vi "CenterFinderUsing2Points.vi"(0 "Operation":enum16{"Manual", "DrawCircle", "Automatic"}(ring)=enum."DrawCircle", 1 "Zone":enum16{"ZoneA", "ZoneB", "ZoneC", "ZoneD"}(ring), 2 "Autofocus":T3={"Enable"=TRUE, "InitialStepSize"=0.05, "Tolerance"=0.02, "Abort"=FALSE} {"Tolerance" format="%#_13g"}, 5 "Component":enum16{"BP", "Si", "HB", "HBonBP", "Other"}(ring), 7 "StopJoyStick":bool, 9 "VisibilityInCamera":enum16{"JoyStick", "AllVisible"}(ring)=enum."AllVisible", 11 "error in (no error)":errorcluster, 12 "Position":enum16{"1", "2"}(ring), 13 "SaveImagesLog":bool=TRUE) -> (4 "Output XYZU":string, 6 "Image":T4(plugin-control), 8 "Image 2":T4[](array[plugin-control]) caption="AllImages", 15 "error out":errorcluster)   [LabVIEW 2021]
uses:
  <vilib>/userDefined/High Color/IMAQdx.ctl
  <vilib>/Analysis/coordinate.llb/2D Cartesian Coordinate Rotation (Scalar).vi
  <vilib>/Analysis/baseanly.llb/Mean (DBL).vi
  include/GlobalVariables.vi
  Other Models/2010/Motion/AbortSingle.vi
  <vilib>/Analysis/NI_AALPro.lvlib
  <vilib>/Analysis/NI_AALBase.lvlib
  <vilib>/vision/driver/NI_Vision_Acquisition_Software.lvlib
panel:
  in  "YoffsetMidFid":dbl=3.5005
  in  "XoffsetMidFid":dbl
  out "DistFids":dbl=50.0
  out "AllMatches":T1(array[cluster]) {"Bounding Box"."y" format="%.2f"; "Bounding Box"."x" format="%.2f"; "Score" format="%.2f"; "Scale" format="%.2f"; "Angle" format="%.2f"; "Position"."y" format="%.2f"; "Position"."x" format="%.2f"}
  in  "Camera":T2="cam1"
  out "OutputFile":string
  out "spreadsheet string 2":string
  out "spreadsheet string":string
  in  "ModuleName":string="T1"
  out "SyringeY":dbl format="%#_7g"
  out "SyringeX":dbl format="%#_7g"
  in  "CamToSyringeYoffset":dbl=126.651
  in  "CamToSyringeXoffset":dbl=167.702
  out "FileUsedForFiducials":string
  out "UsedCoordinates":string
  out "CameraGcode":string
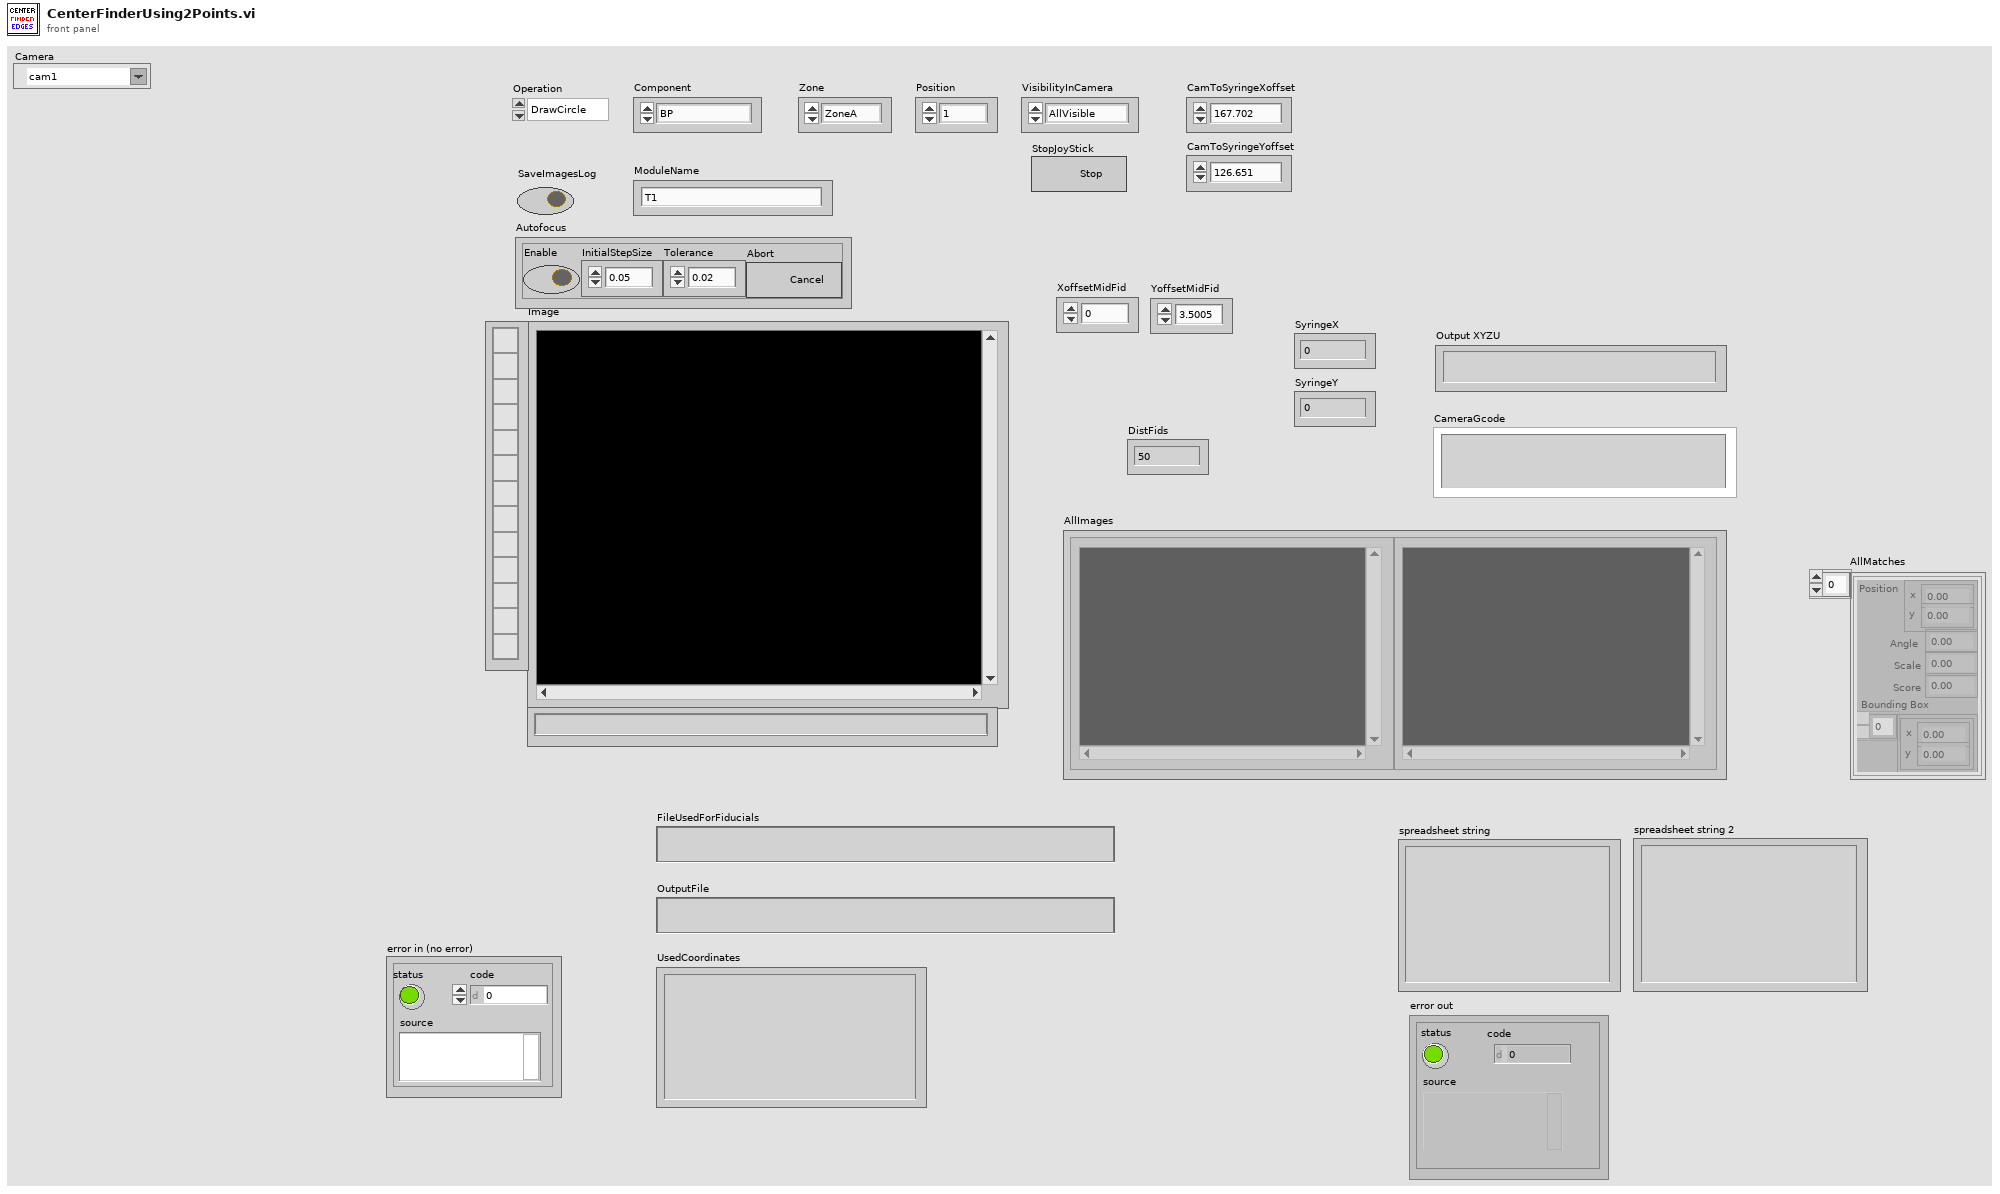
[diagram p1: front panel]
types:
  T1 = cluster{"Position":cluster{"x":sgl, "y":sgl}, "Angle":sgl, "Scale":sgl, "Score":sgl, "Bounding Box":cluster{"x":sgl, "y":sgl}[]}[]
  T2 = typedef "IMAQdx.ctl" = refnum<k21>
  T3 = cluster{"Enable":bool, "InitialStepSize":dbl, "Tolerance":dbl, "Abort":bool}
  T4 = typedef "IMAQ Image.ctl" = refnum<image>
  T5 = cluster{"Number of Matches Requested":i32, "Minimum Match Score":sgl, "Angle Ranges":cluster{"Start Angle":sgl, "End Angle":sgl}[]}
  T6 = typedef "Image Type" = u32
  T7 = typedef "IMAQ Point" = cluster{"X":sgl, "Y":sgl}
  T8 = typedef "IMAQ Circle" = cluster{"Center X":i32, "Center Y":i32, "Inner Radius":i32, "Outer Radius":i32, "Start Angle":dbl, "End Angle":dbl}
  T9 = enum16{"Left Button", "Center Button", "Right Button", "Window Close"}
  T10 = enum16{"open", "replace", "create", "open or create", "replace or create", "replace or create with confirmation"}
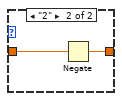
[diagram p2: hidden frame]
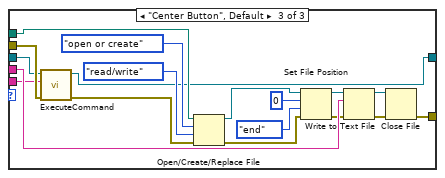
[diagram p5: hidden frame]
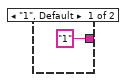
[diagram p6: hidden frame]
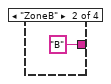
[diagram p7: hidden frame]
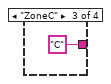
[diagram p8: hidden frame]
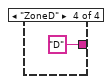
[diagram p9: hidden frame]
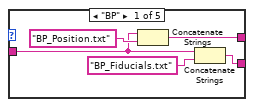
[diagram p10: hidden frame]
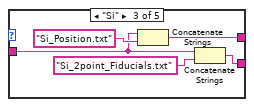
[diagram p11: hidden frame]
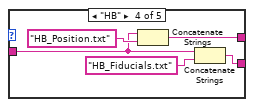
[diagram p12: hidden frame]
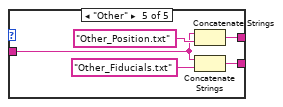
[diagram p13: hidden frame]
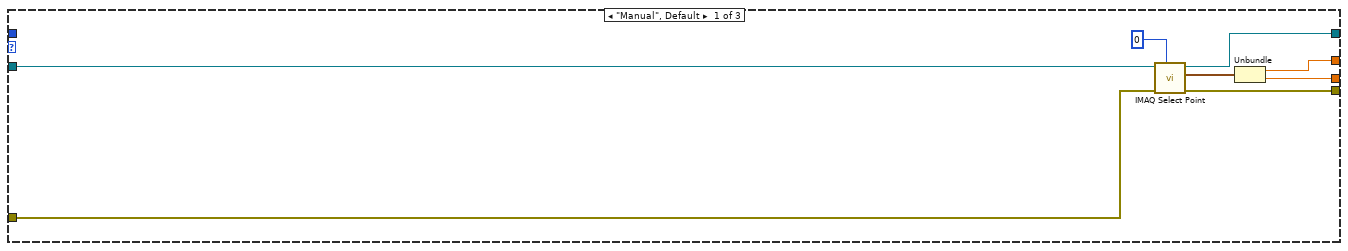
[diagram p14: hidden frame]
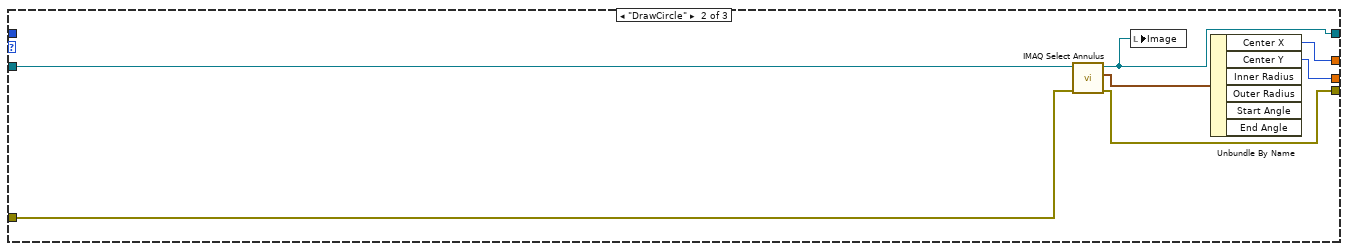
[diagram p15: hidden frame]
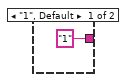
[diagram p17: hidden frame]
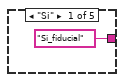
[diagram p18: hidden frame]
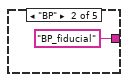
[diagram p19: hidden frame]
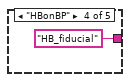
[diagram p20: hidden frame]
diagram:
  w49 = "%f" ("format string")
  w87 = "\t"
  w84 = i16 6 ("width (-)")
  # "Write the XYZU of the baseplate to a text file & move the gantry?"
  # "Prepare to move the gantry to see the center of baseplate in camera."
  # "AllVisble: Assumes that you know the coordinates of all corners (fiducials) well. No need for any adjustments.\nJoyStick: Use joystick at each point to make good image.\nClickMove: Use \"AdjustCamera\" panel and move the gantry stepwise. Click \"Done\" when you're satisfied with the picture."
  n1 = flat-sequence {
    tunnel: [w96] -> w45
    tunnel: w45 -> [w112]
    tunnel: [w111] -> w44
    tunnel: [w110] -> w42
    tunnel: [w109] -> w39
    tunnel: w44 -> [w164]
    tunnel: [w164] -> w43
    tunnel: w42 -> [w157]
    tunnel: [w152] -> w41
    tunnel: [w163] -> w40
    tunnel: w39 -> [w162]
    tunnel: [w162] -> w38
    tunnel: [w156] -> w30
    tunnel: [w155] -> w29
    tunnel: 2 -> [w191]
    tunnel: "VisibilityInCamera" -> [w184]
    tunnel: w43 -> [w182]
    tunnel: w41 -> [w174]
    tunnel: w40 -> [w181]
    tunnel: w38 -> [w180]
    tunnel: w30 -> [w172]
    tunnel: w29 -> [w173]
    tunnel: [w190] -> w28
    tunnel: [w189] -> w27
    tunnel: [w188] -> w26
    tunnel: [w187] -> w25
    tunnel: [w186] -> w24
    tunnel: [w185] -> w23
    tunnel: [w183] -> w22
    tunnel: [w180] -> w21
    tunnel: [w179] -> w20
    tunnel: [w171] -> w19
    tunnel: [w468] -> w36
    tunnel: [w469] -> w37
    tunnel: [w470] -> w54
    tunnel: [w471] -> w15
    tunnel: [w465] -> w16
    tunnel: [w472] -> _
    tunnel: [w473] -> w91
    tunnel: [w474] -> w50
    tunnel: [w475] -> w51
    tunnel: w28 -> [w475]
    tunnel: w27 -> [w474]
    tunnel: w26 -> [w473]
    tunnel: w25 -> [w472]
    tunnel: w24 -> [w466]
    tunnel: w23 -> [w471]
    tunnel: w22 -> [w470]
    tunnel: w21 -> [w469]
    tunnel: w20 -> [w468]
    tunnel: w19 -> [w467]
    frame #0 {
      n2 = case shown="\"ZoneA\", Default" "Zone" {
        tunnel: ["A" "B" "C" "D"] -> w100
        frame "ZoneA", Default {
        }
        frame "ZoneB" {
        }
        frame "ZoneC" {
        }
        frame "ZoneD" {
        }
      }
      n3 = case shown="\"2\"" "Position" {
        tunnel: ["1" "2"] -> w101
        frame "1", Default {
        }
        frame "2" {
        }
      }
      n4 = Concatenate Strings(w100, w101, "_" ("string")) -> (w96:string)
      "UsedCoordinates" <- ""
    }
    frame #1 {
      n5 = Concatenate Strings("C:\\Users\\TTUHEP\\Documents\\LabVIEW\\GantryPrograms\\", "Configs\\" ("string"), w112) -> (w119:string)
      n6 = case shown="\"HBonBP\"" "Component" {
        tunnel: w119 -> [w127 w132 w138 w143 w148]
        tunnel: [w128 w133 w140 w145 w150] -> w122
        tunnel: [w129 w134 w137 w142 w147] -> w109
        frame "BP" {
          n7 = Concatenate Strings(w127, "BP_Position.txt") -> (w129:string)
          n8 = Concatenate Strings(w127, "BP_Fiducials.txt") -> (w128:string)
        }
        frame "HBonBP" {
          n9 = Concatenate Strings(w132, "BP_Position.txt") -> (w134:string)
          n10 = Concatenate Strings(w132, "HBonBP_Fiducials.txt") -> (w133:string)
        }
        frame "Si" {
          n11 = Concatenate Strings(w138, "Si_Position.txt") -> (w137:string)
          n12 = Concatenate Strings(w138, "Si_2point_Fiducials.txt") -> (w140:string)
        }
        frame "HB" {
          n13 = Concatenate Strings(w143, "HB_Position.txt") -> (w142:string)
          n14 = Concatenate Strings(w143, "HB_Fiducials.txt") -> (w145:string)
        }
        frame "Other" {
          n15 = Concatenate Strings(w148, "Other_Position.txt") -> (w147:string)
          n16 = Concatenate Strings(w148, "Other_Fiducials.txt") -> (w150:string)
        }
      }
      "FileUsedForFiducials" <- w122
      "OutputFile" <- w109
      n17 = String To Path(string=w122) -> (path=w120:path)
      n18 = Concatenate Strings("This file does not exist:" ("ErrorMessage"), w122) -> (w123:string)
      n19 = call <vilib>:"Check if File or Folder Exists.vi"("error in (no error)"="error in (no error)", "path"=w120) -> ("error out"=w121:errorcluster, "file or folder exists?"=w124:bool, "dup path"=w111:path)  [unwired: 7 in]
      n20 = Not(x=w124) -> (.not. x?=w125:bool)
      n21 = call "AddError.vi"("NoErrorMessage"="InFile OK", "ErrorMessage"=w123, "error in"=w121, "code"=-995, "Error?"=w125) -> ("Error out"=w110:errorcluster)  [unwired: 6 in]
    }
    frame #2 {
      w158 = T6 0 items=["Grayscale (U8)", "Grayscale (I16)", "Grayscale (SGL)", "Complex (CSG)", "RGB (U32)", "HSL (U32)", "RGB (U64)", "Grayscale (U16)"] ("Image Type")
      # "Set the size of the window while selecting the point."
      n22 = call "IMAQ WindSize"("Scrollbars? (N)"=TRUE, "Width & Height"=cluster{"Width":i32, "Height":i32} {"Width"=1333, "Height"=1000}, "Window Number"=0) -> ()  [unwired: 3 in, 3 out]
      n23 = call "IMAQ Create"("Image Name"="name1" ("ImageName"), "Image Type"=w158, "error in (no error)"=w157) -> ("New Image"=w155:T4, "error out"=w160:errorcluster)  [unwired: 2 in]
      n24 = call "Connect.vi"("error in (no error)"=w157) -> ("error out"=w166:errorcluster, "controller"=w167:refnum<k24>)  [unwired: 9 in]
      n25 = call "ExecuteCommand.vi"("error in (no error)"=w166, "Command Code"="G90\nG1 Z0 F100", "controller in"=w167) -> ("error out"=w154:errorcluster, "controller out"=w163:refnum<k24>)  [unwired: 6 in, 1 out]
      n26 = call <vilib>:"IMAQdx Open Camera.vi"("error in"=w160, "Session In"="Camera") -> ("error out"=w153:errorcluster, "Session Out"=w156:T2)  [unwired: 8 in]
      n27 = Merge Errors(w154, w153) -> (w152:errorcluster)
    }
    frame #3 {
      n28 = local read "Autofocus"() -> (w178:T3)
      n29 = local read "Autofocus"() -> (w176:T3)
      n30 = Unbundle By Name(w178) -> ("Enable"=w177:bool)
      n31 = Unbundle By Name(w176) -> ("Abort"=w175:bool)
      n32 = for {
        N: w191 -> [_]
        tunnel: w181 -> [w251]
        tunnel: w182 -> [w234]
        tunnel: [w232] -> w190 mode=indexing
        tunnel: [w231] -> w189 mode=indexing
        tunnel: [w230] -> w188 mode=indexing
        tunnel: [w226] -> w187 mode=indexing
        tunnel: [w225] -> w185
        tunnel: w184 -> [w224]
        tunnel: w175 -> [w223]
        tunnel: w177 -> [w222]
        tunnel: [w218] -> w183
        tunnel: [w213] -> w179 mode=indexing
        shift-right: [w216] -> w186
        shift-left: w174 -> [w200]
        tunnel: w173 -> [w199]
        shift-right: [w193] -> w171
        shift-left: w172 -> [w192]
        i -> [w211]
        w202 = T6 6 items=["Grayscale (U8)", "Grayscale (I16)", "Grayscale (SGL)", "Complex (CSG)", "RGB (U32)", "HSL (U32)", "RGB (U64)", "Grayscale (U16)"] ("Image Type")
        # "Array of XY cluser"
        # "Z array"
        # "Y array"
        # "X array"
        # "Read text file line by line. Each line contains X,Y,Z coordinates for the gantry."
        n33 = call "GetArrayFmTxtFile.vi"("error in"=w200, "LineNo."=w211, "TextFile"=w234) -> ("error out"=w233:errorcluster, "Array"=w258:dbl[])
        n34 = Index Array(array=w258, index=0) -> (element=w253:dbl)
        n35 = Index Array(array=w258, index=1) -> (element=w252:dbl)
        n36 = Index Array(array=w258, index=2) -> (element=w254:dbl)
        n37 = call "Move.vi"("X"=w253, "Absolute"=TRUE, "Y"=w252, "Z"=w254, "SpeedXY (mm/s)"=100.0, "SpeedZ (mm/s)"=100.0, "Move Z first"=FALSE) -> ("Position Gcode"=w250:string)  [unwired: 8 in]
        n38 = call "ExecuteCommand.vi"("error in (no error)"=w233, "Command Code"=w250, "controller in"=w251) -> ("error out"=w198:errorcluster, "controller out"=w249:refnum<k24>)  [unwired: 6 in, 1 out]
        n39 = call <vilib>:"IMAQdx Snap2.vi"("error in"=w198, "Image In"=w199, "Session In"=w192) -> ("error out"=w197:errorcluster, "Image Out"=w195:T4, "Session Out"=w196:T2)  [unwired: 6 in]
        n40 = local write "Image"(w195) -> ()
        n41 = case shown="\"JoyStick\", Default" w224 {
          tunnel: w196 -> [w372 w434]
          tunnel: w249 -> [w390 w446]
          tunnel: w197 -> [w388 w447]
          tunnel: [w368 w435] -> w220
          tunnel: [w377 w441] -> w238
          tunnel: [w378 w439] -> w194
          tunnel: w223 -> [w381 w444]
          tunnel: w222 -> [w375 w445]
          tunnel: "name1" ("ImageName") -> [w374 w433]
          tunnel: w195 -> [w371 w432]
          tunnel: [w367 w431] -> w193
          frame "JoyStick", Default {
            # "Use joystick to go to a position where camera sees good image."
            n42 = while {
              tunnel: [w418] -> w369
              tunnel: w390 -> [w424]
              tunnel: [w423] -> w386
              tunnel: [w422] -> w387
              tunnel: w388 -> [w417]
              tunnel: w372 -> [w415]
              tunnel: w371 -> [w414]
              tunnel: [w413] -> w370
              stop <- w419 stop-if-true
              n43 = call <vilib>:"IMAQdx Snap2.vi"("error in"=w417, "Image In"=w414, "Session In"=w415) -> ("error out"=w416:errorcluster, "Image Out"=w418:T4, "Session Out"=w413:T2)  [unwired: 6 in]
              n44 = local write "Image"(w418) -> ()
              n45 = global read "GlobalVariables.vi" "StopJoyStick"() -> (w420:bool)
              n46 = Or(x="StopJoyStick", y=w420) -> (x .or. y?=w419:bool)
              n47 = case shown="False" w419 {
                tunnel: w424 -> [w426 w430]
                tunnel: w416 -> [w425 w429]
                tunnel: [w425 w428] -> w423
                tunnel: [w426 w427] -> w422
                frame False {
                }
                frame True {
                  n48 = call-poly "Abort.vi"("error in (no error)"=w429, "controller in"=w430) -> ("error out"=w428:errorcluster, "controller out"=w427:refnum<k24>)  [unwired: 8 in]
                }
              }
            }
            n49 = global write "GlobalVariables.vi" "StopJoyStick"(FALSE ("StopJoyStick")) -> ()
            n50 = call "ExecuteCommand.vi"("error in (no error)"=w388, "Command Code"="JOYSTICK 2D RESET\nJOYSTICK 2D AXISGROUP 1 Y X\nJOYSTICK 2D AXISGROUP 2 Y Z\nJOYSTICK 2D ON", "controller in"=w390) -> ("error out"=w389:errorcluster)  [unwired: 6 in, 2 out]
            n51 = call <vilib>:"Clear Errors.vi"("error in (no error)"=w389) -> ()  [unwired: 5 in, 2 out]
            n52 = call "GetGantryPosition.vi"("error in (no error)"=w386, "Controller In"=w387) -> ("error out"=w382:errorcluster, "controller out"=w380:refnum<k24>, "Position_XYZ"=w376:string)  [unwired: 3 in, 4 out]
            n53 = case shown="False" w375 {
              tunnel: w382 -> [w396 w412]
              tunnel: w381 -> [_ w405]
              tunnel: w380 -> [w394 w406]
              tunnel: [w395 w410] -> w379
              tunnel: [w396 w409] -> w378
              tunnel: [w394 w408] -> w377
              tunnel: w376 -> [w395 _]
              tunnel: w374 -> [_ _]
              tunnel: w370 -> [w392 w400]
              tunnel: w369 -> [w393 w399]
              tunnel: [w393 w398] -> w368
              tunnel: [w392 w397] -> w367
              frame False {
              }
              frame True {
                n54 = local read "Autofocus"() -> (w403:T3)
                n55 = Unbundle By Name(w403) -> ("InitialStepSize"=w401:dbl, "Tolerance"=w402:dbl)
                n56 = call "Autofocus.vi"("controller in"=w406, "AbortAutoFocus"=w405, "ImageIn"=w399, "SafeMaxZ"=80.0, "InitialStepSize"=w401, "Tolerance"=w402, "error in (no error)"=w412, "SessionIn"=w400) -> ("controller out"=w411:refnum<k24>, "Image"=w398:T4, "Session Out"=w397:T2, "error out"=w407:errorcluster)  [unwired: 2 in, 2 out]
                n57 = local write "Image"(w398) -> ()
                n58 = call "GetGantryPosition.vi"("error in (no error)"=w407, "Controller In"=w411) -> ("error out"=w409:errorcluster, "controller out"=w408:refnum<k24>, "Position_XYZ"=w410:string)  [unwired: 3 in, 4 out]
              }
            }
            n59 = local read "UsedCoordinates"() -> (w384:string)
            n60 = Concatenate Strings(w384, "\r", w379) -> (w385:string)
            n61 = local write "UsedCoordinates"(w385) -> ()
          }
          frame "AllVisible" {
            # "No need to move gantry to take a good pic."
            n62 = case shown="False" w445 {
              tunnel: w444 -> [_ w459]
              tunnel: [w451 w462] -> w440
              tunnel: [w450 w464] -> w442
              tunnel: w447 -> [w451 w463]
              tunnel: w446 -> [w450 w461]
              tunnel: [w449 w458] -> w435
              tunnel: w434 -> [w448 w454]
              tunnel: w433 -> [_ _]
              tunnel: w432 -> [w449 w453]
              tunnel: [w448 w452] -> w431
              frame False {
              }
              frame True {
                n63 = local read "Autofocus"() -> (w457:T3)
                n64 = Unbundle By Name(w457) -> ("InitialStepSize"=w456:dbl, "Tolerance"=w455:dbl)
                n65 = call "Autofocus.vi"("controller in"=w461, "AbortAutoFocus"=w459, "ImageIn"=w453, "SafeMaxZ"=80.0, "InitialStepSize"=w456, "Tolerance"=w455, "error in (no error)"=w463, "SessionIn"=w454) -> ("controller out"=w464:refnum<k24>, "Image"=w458:T4, "Session Out"=w452:T2, "error out"=w462:errorcluster)  [unwired: 2 in, 2 out]
                n66 = local write "Image"(w458) -> ()
              }
            }
            n67 = local read "UsedCoordinates"() -> (w437:string)
            n68 = call "GetGantryPosition.vi"("error in (no error)"=w440, "Controller In"=w442) -> ("error out"=w439:errorcluster, "controller out"=w441:refnum<k24>, "Position_XYZ"=w438:string)  [unwired: 3 in, 4 out]
            n69 = Concatenate Strings(w437, "\r", w438) -> (w436:string)
            n70 = local write "UsedCoordinates"(w436) -> ()
          }
        }
        n71 = case shown="\"Automatic\"" "Operation" {
          tunnel: [w267 w274 w285] -> w246
          tunnel: [w266 w273 w284] -> w245
          tunnel: [w265 w275 w293] -> w244
          tunnel: w194 -> [w264 w270 w309]
          tunnel: w220 -> [w263 w272 w314]
          tunnel: w211 -> [_ _ _]
          tunnel: [w262 w271 w291] -> w212
          frame "Manual", Default {
            n72 = call "IMAQ Select Point"("Window Number (0...15)"=0, "error in (no error)"=w264, "Image In"=w263) -> ("error out"=w265:errorcluster, "Point"=w268:T7, "Image Out (duplicate)"=w262:T4)  [unwired: 5 in, 1 out]
            n73 = Unbundle(w268) -> ("X"=w267:sgl, "Y"=w266:sgl)
          }
          frame "DrawCircle" {
            n74 = call "IMAQ Select Annulus"("error in (no error)"=w270, "Image In"=w272) -> ("error out"=w275:errorcluster, "Annulus"=w276:T8, "Image Out (duplicate)"=w271:T4)  [unwired: 6 in, 1 out]
            n75 = local write "Image"(w271) -> ()
            n76 = Unbundle By Name(w276) -> ("Center X"=w274:i32, "Center Y"=w273:i32)  [unwired: 4 out]
          }
          frame "Automatic" {
            w289 = sgl 50.0 ("y")
            w307 = ""
            n77 = local read "Position"() -> (w296:enum16{"1", "2"})
            n78 = case shown="\"2\"" w296 {
              tunnel: ["1" "2"] -> w295
              frame "1", Default {
              }
              frame "2" {
              }
            }
            n79 = local read "Component"() -> (w311:enum16{"BP", "Si", "HB", "HBonBP", "Other"})
            n80 = case shown="\"HB\"" w311 {
              tunnel: ["Si_fiducial" "BP_fiducial" "HB_fiducial" "HB_fiducial" "Other_fiducial"] -> w310
              tunnel: w295 -> [_ _ _ _ _]
              frame "Si" {
              }
              frame "BP" {
              }
              frame "HB" {
              }
              frame "HBonBP" {
              }
              frame "Other" {
              }
            }
            n81 = Concatenate Strings("Could not parse/find this template file for pattern recognition:" ("ErrorMessage"), w310) -> (w302:string)
            n82 = call "JSONfileReader.vi"("error in"=w309, "Variant"=w307, "ItemName"=w310, "FileIn"=path "C:/Users/TTUHEP/Documents/LabVIEW/GantryPrograms/Configs/PatternRecognTemplateMaps.json" ("PatterRecognTemplateMap")) -> ("error out"=w299:errorcluster, "Data"=w308:variant, "Found"=w305:bool)
            n83 = Not(x=w305) -> (.not. x?=w304:bool)
            n84 = Variant To Data(error in=w299, type=w307, Variant=w308) -> (data=w306:string, error out=w298:errorcluster)
            n85 = call "AddError.vi"("NoErrorMessage"="Template file name found from json.", "ErrorMessage"=w302, "error in"=w298, "code"=-902, "Error?"=w304) -> ("Error out"=w297:errorcluster)  [unwired: 6 in]
            n86 = call "PatternRecognition.vi"("error in (no error)"=w297, "MatchParameters"=T5 {"Number of Matches Requested"=1, "Minimum Match Score"=500.0, "Angle Ranges"=[{"Start Angle"=0.0, "End Angle"=0.0}]}, "ImageIn"=w314, "TemplateFileName"=w306) -> ("error out"=w280:errorcluster, "AllMatches"=→"AllMatches":T1, "Position"=w313:cluster{"x":sgl, "y":sgl}, "ImageFoundPattern"=w292:T4, "Number of Matches"=w294:i32)  [unwired: 2 in]
            n87 = Equal To 0?(x=w294) -> (x = 0?=w290:bool)
            n88 = Unbundle(w313) -> ("x"=w283:sgl, "y"=w282:sgl)
            n89 = call <vilib>:"Clear Errors.vi"("error in (no error)"=w280, "specific error code to clear (0: all)"=-903) -> ("error out"=w279:errorcluster)  [unwired: 4 in, 1 out]
            n90 = Less?(x=w283, y=w289) -> (x < y?=w288:bool)
            n91 = Less?(x=w282, y=w289) -> (x < y?=w287:bool)
            n92 = Compound Arithmetic op=OR(w290, w288, w287) -> (w286:bool)
            n93 = case shown="True" w286 {
              tunnel: w279 -> [w318 w325]
              tunnel: [w318 w324] -> w293
              tunnel: w292 -> [w317 w323]
              tunnel: [w317 w322] -> w291
              tunnel: [w316 w320] -> w285
              tunnel: [w315 w319] -> w284
              tunnel: w283 -> [w316 _]
              tunnel: w282 -> [w315 _]
              frame False {
              }
              frame True {
                n94 = call "IMAQ Select Annulus"("Window Number (0...15)"=0, "error in (no error)"=w325, "Image In"=w323) -> ("error out"=w324:errorcluster, "Annulus"=w321:T8, "Image Out (duplicate)"=w322:T4)  [unwired: 5 in, 1 out]
                n95 = Unbundle(w321) -> ("Center X"=w320:i32, "Center Y"=w319:i32)  [unwired: 4 out]
              }
            }
          }
        }
        n96 = Number To Decimal String(number=w211) -> (decimal integer string=w210:string)  [unwired: 1 in]
        n97 = Concatenate Strings("imgTemp" ("string"), w210) -> (w207:string)
        n98 = call "GetPixelToGantryRelPosition.vi"("error in (no error)"=w244, "PixelY"=w245, "PixelX"=w246) -> ("error out"=w205:errorcluster, "YmmRelGH"=w242:dbl, "XmmRelGH"=w243:dbl)
        n99 = call "IMAQ Create"("Image Name"=w207, "Image Type"=w202, "error in (no error)"=w205) -> ("New Image"=w206:T4, "error out"=w204:errorcluster)  [unwired: 2 in]
        n100 = call "IMAQ Copy"("error in (no error)"=w204, "Image Dst"=w206, "Image Src"=w212) -> ("error out"=w203:errorcluster, "Image Dst Out"=w208:T4)  [unwired: 3 in]
        n101 = Build Array(w208) -> (w213:T4[])
        n102 = flat-sequence {
          tunnel: w203 -> [w358]
          tunnel: [w358] -> w248
          tunnel: w238 -> [w357]
          tunnel: [w357] -> w247
          tunnel: [w366] -> w217
          tunnel: [w365] -> w241
          tunnel: [w364] -> w240
          tunnel: [w363] -> w225
          tunnel: [w362] -> w239
          tunnel: w248 -> [w361]
          tunnel: w247 -> [w360]
          frame #0 {
            n103 = Wait (ms)(milliseconds to wait=u32 1000) -> ()  [unwired: 1 out]
          }
          frame #1 {
            n104 = call "GetGantryPosition.vi"("error in (no error)"=w361, "Controller In"=w360) -> ("error out"=w366:errorcluster, "Position Y"=w365:dbl, "Position X"=w364:dbl, "controller out"=w363:refnum<k24>, "Position Z"=w362:dbl)  [unwired: 3 in, 2 out]
          }
        }
        n105 = Add(x=w243, y=w240) -> (x+y=w237:dbl)
        n106 = Add(x=w242, y=w241) -> (x+y=w236:dbl)
        n107 = case shown="True" "SaveImagesLog" {
          tunnel: w212 -> [w334 w352]
          tunnel: w211 -> [_ w350]
          tunnel: ["" w342] -> w218
          tunnel: w217 -> [w335 w341]
          tunnel: [w335 w340] -> w216
          tunnel: [w334 w339] -> w201
          frame False {
          }
          frame True {
            w344 = "C:\\Users\\TTUHEP\\Documents\\LabVIEW\\GantryPrograms\\LogFiles\\CalibrationData\\"
            n108 = local read "Component"() -> (w338:enum16{"BP", "Si", "HB", "HBonBP", "Other"})
            n109 = case shown="\"HB\"" w338 {
              tunnel: ["BP_fiducial" "Si_fiducial" "Other_fiducial" "HB_fiducial"] -> w337
              frame "BP" {
              }
              frame "Si", Default {
              }
              frame "Other" {
              }
              frame "HB" {
              }
            }
            n110 = Number To Decimal String(number=w350) -> (decimal integer string=w348:string)  [unwired: 1 in]
            n111 = Concatenate Strings(w344, "ModuleName") -> (w342:string)
            n112 = Concatenate Strings(w344, "ModuleName", w337, "Image" ("string"), w348, ".png" ("string")) -> (w346:string)
            n113 = String To Path(string=w346) -> (path=w345:path)
            n114 = call-poly "IMAQ Write File 2"("error in (no error)"=w341, "Image Quality"=u32 1000, "File Path"=w345, "Image"=w352) -> ("error out"=w340:errorcluster, "Image Out (duplicate)"=w339:T4)  [unwired: 6 in]
          }
        }
        "Image" <- w201
        n115 = call-poly <vilib>:"2D Cartesian Coordinate Rotation.vi"("theta"=0.0, "y"=w236, "x"=w237) -> ("y out"=w228:dbl, "x out"=w229:dbl)  [unwired: 6 in, 1 out]
        n116 = Bundle("x out"=w229, "y out"=w228) -> (w227:cluster{"x out":dbl, "y out":dbl})  [unwired: 1 in]
        n117 = global write "GlobalVariables.vi" "Image"(w201) -> ()
        n118 = Build Array(w227) -> (w226:cluster{"x out":dbl, "y out":dbl}[])
        n119 = Build Array(w229) -> (w232:dbl[])
        n120 = Build Array(w228) -> (w231:dbl[])
        n121 = Build Array(w239) -> (w230:dbl[])
      }
    }
    frame #4 {
      n122 = call <vilib>:"IMAQdx Close Camera.vi"("error in"=w466, "Session In"=w467) -> ("error out"=w465:errorcluster)  [unwired: 9 in]
    }
  }
  n123 = Array To Spreadsheet String(array=w51, 3:w49) -> (spreadsheet string=→"spreadsheet string":string)  [unwired: 1 in]
  n124 = Array To Spreadsheet String(array=w50, 3:w49) -> (spreadsheet string=→"spreadsheet string 2":string)  [unwired: 1 in]
  n125 = String To Path(string=w37) -> (path=w46:path)
  n126 = Index Array(array=w36, index (col)=0 ("disabled index (col)")) -> (element=→"Image 2":T4[])  [unwired: 1 in]
  n127 = Index Array "X"(array=w51, index (col)=0 ("disabled index (col)")) -> (element=w18:dbl[])  [unwired: 1 in]
  n128 = Index Array "Y"(array=w50, index (col)=0 ("disabled index (col)")) -> (element=w17:dbl[])  [unwired: 1 in]
  n129 = Index Array "Z"(array=w91, index (col)=0 ("disabled index (col)")) -> (element=w90:dbl[])  [unwired: 1 in]
  n130 = formula code="float64 xMid = 0.5*(xin[0]+xin[1]);\nfloat64 yMid = 0.5*(yin[0]+yin[1]);\nfloat64 dist = sqrt((xin[0]-xin[1])*(xin[0]-xin[1]) + (yin[0]-yin[1])*(yin[0]-yin[1]));\nfloat64 angle = 90.0 - (asin(abs(yin[0] - yin[1])/dist)*180.0/3.14159);\nif((xin[0]-xin[1])/(yin[0]-yin[1]) <=0)\n  angle = angle;\nelse\n  angle = -angle;"("xin"=w18, "yin"=w17) -> ("xMid"=w11:dbl, "yMid"=w7:dbl, "angle"=w4:dbl, "dist"=→"DistFids":dbl)
  n131 = local read "Position"() -> (w3:enum16{"1", "2"})
  n132 = case shown="\"1\", Default" w3 {
    tunnel: "YoffsetMidFid" -> [w476 w478]
    tunnel: [w476 w477] -> w1
    frame "1", Default {
    }
    frame "2" {
      n133 = Negate(x=w478) -> (-x=w477:dbl)
    }
  }
  n134 = Negate(x=w4) -> (-x=w5:dbl)
  n135 = call-poly <vilib>:"Mean.vi"("X"=w90) -> ("mean"=w67:dbl)  [unwired: 1 out]
  n136 = expression code="(x/180.0)*pi" "degrees to radians"(w5) -> (w12:dbl)
  n137 = call-poly <vilib>:"2D Cartesian Coordinate Rotation.vi"("theta"=w12, "y"=w1, "x"="XoffsetMidFid") -> ("y out"=w8:dbl, "x out"=w10:dbl)  [unwired: 6 in, 1 out]
  n138 = Add(x=w7, y=w8) -> (x+y=w6:dbl)
  n139 = Add(x=w11, y=w10) -> (x+y=w9:dbl)
  n140 = Number To Fractional String(number=w6, precision (6)=w84) -> (F-format string=w88:string)  [unwired: 2 in]
  n141 = Number To Fractional String(number=w9, precision (6)=w84) -> (F-format string=w89:string)  [unwired: 2 in]
  n142 = Number To Fractional String(number=w67, precision (6)=w84) -> (F-format string=w83:string)  [unwired: 2 in]
  n143 = call "CameraXYusingGantryHeadXY.vi"("GantryY"=w6, "GantryX"=w9) -> ("CamY"=w60:dbl, "CamX"=w62:dbl)
  n144 = Number To Fractional String(number=w4, precision (6)=i16 4 ("width (-)")) -> (F-format string=w85:string)  [unwired: 2 in]
  n145 = call "Move.vi"("X"=w62, "Absolute"=TRUE, "Y"=w60, "Z"=w67, "SpeedXY (mm/s)"=100.0, "SpeedZ (mm/s)"=50.0, "Move Z first"=TRUE) -> ("Position Gcode"=w70:string)  [unwired: 8 in]
  "CameraGcode" <- w70
  n146 = Add(x="CamToSyringeYoffset", y=w60) -> (x+y=→"SyringeY":dbl)
  n147 = Concatenate Strings(w89, w87, w88, w87, w83, w87, w85, "\r") -> (w81:string)
  "Output XYZU" <- w81
  n148 = Add(x="CamToSyringeXoffset", y=w62) -> (x+y=→"SyringeX":dbl)
  n149 = Concatenate Strings("Overwrite/Append ", w81, " to file ", w37, " ?" ("string")) -> (w78:string)
  n150 = call <vilib>:"Three Button Dialog.vi"("Right Button Text (\"Cancel\")"="Do nothing" ("Right Button Text (\"Cancel\")"), "Center Button Text (\"No\")"="Append" ("Center Button Text (\"No\")"), "Left Button Text (\"Yes\")"="Overwrite" ("Left Button Text (\"Yes\")"), "message"=w78) -> ("Which Button?"=w77:T9)  [unwired: 7 in]
  n151 = case shown="\"Left Button\"" w77 {
    tunnel: w81 -> [w486 _ w508]
    tunnel: w46 -> [w485 _ w507]
    tunnel: w16 -> [w484 w494 w506]
    tunnel: w70 -> [w483 _ w505]
    tunnel: w15 -> [w482 w493 w504]
    tunnel: [w479 w494 w495] -> w56
    tunnel: [w481 w493 w503] -> w69
    frame "Left Button" {
      n152 = call "ExecuteCommand.vi"("error in (no error)"=w484, "Command Code"=w483, "controller in"=w482) -> ("error out"=w480:errorcluster, "controller out"=w481:refnum<k24>)  [unwired: 6 in, 1 out]
      n153 = Open/Create/Replace File(file path (use dialog)=w485, error in=w480, operation (0:open)=T10."replace or create", access (0:read/write)=enum16{"read/write", "read-only", "write-only"}."read/write") -> (refnum out=w492:refnum<file>, error out=w489:errorcluster)  [unwired: 2 in, 1 out]
      n154 = Write to Text File(file (use dialog)=w492, text=w486, error in=w489) -> (refnum out=w487:refnum<file>, error out=w488:errorcluster)  [unwired: 1 in, 1 out]
      n155 = Close File(refnum=w487, error in=w488) -> (error out=w479:errorcluster)  [unwired: 1 out]
    }
    frame "Right Button" {
    }
    frame "Center Button", Default {
      n156 = call "ExecuteCommand.vi"("error in (no error)"=w506, "Command Code"=w505, "controller in"=w504) -> ("error out"=w496:errorcluster, "controller out"=w503:refnum<k24>)  [unwired: 6 in, 1 out]
      n157 = Open/Create/Replace File(file path (use dialog)=w507, error in=w496, operation (0:open)=T10."open or create", access (0:read/write)=enum16{"read/write", "read-only", "write-only"}."read/write") -> (refnum out=w500:refnum<file>, error out=w498:errorcluster)  [unwired: 2 in, 1 out]
      n158 = Set File Position(offset (in bytes) (0)=i64 0, refnum=w500, from (0:start)=enum16{"start", "end", "current"}."end", error in=w498) -> (refnum out=w499:refnum<file>, error out=w497:errorcluster)
      n159 = Write to Text File(file (use dialog)=w499, text=w508, error in=w497) -> (refnum out=w509:refnum<file>, error out=w510:errorcluster)  [unwired: 1 in, 1 out]
      n160 = Close File(refnum=w509, error in=w510) -> (error out=w495:errorcluster)  [unwired: 1 out]
    }
  }
  n161 = call "CaptureImage.vi"("Camera"=T2 "cam1", "ImageName"="CurrImage", "Draw50MicroCircleAtCenter"=TRUE, "error in (no error)"=w56) -> ("Image"=w33:T4, "error out"=w55:errorcluster)  [unwired: 3 in]
  n162 = local write "Image"(w33) -> ()
  n163 = global write "GlobalVariables.vi" "Image"(w33) -> ()
  n164 = call "Disconnect.vi"("error in (no error)"=w55, "controller"=w69) -> ("error out"=w52:errorcluster)  [unwired: 9 in]
  n165 = local read "SaveImagesLog"() -> (w57:bool)
  n166 = case shown="True" w57 {
    tunnel: w52 -> [w513 w528]
    tunnel: w54 -> [_ w521]
    tunnel: w33 -> [_ w516]
    tunnel: [w513 w514] -> w53
    frame False {
    }
    frame True {
      n167 = Concatenate Strings(w521, "UsedXYZ.txt") -> (w526:string)
      n168 = local read "UsedCoordinates"() -> (w523:string)
      n169 = Concatenate Strings(w521, "CenterImage.png") -> (w519:string)
      n170 = String To Path(string=w526) -> (path=w525:path)
      n171 = String To Path(string=w519) -> (path=w517:path)
      n172 = Open/Create/Replace File(file path (use dialog)=w525, error in=w528, operation (0:open)=T10."open or create", access (0:read/write)=enum16{"read/write", "read-only", "write-only"}."read/write") -> (refnum out=w524:refnum<file>, error out=w532:errorcluster)  [unwired: 2 in, 1 out]
      n173 = Write to Text File(file (use dialog)=w524, text=w523, error in=w532) -> (refnum out=w522:refnum<file>, error out=w531:errorcluster)  [unwired: 1 in, 1 out]
      n174 = Close File(refnum=w522, error in=w531) -> (error out=w515:errorcluster)  [unwired: 1 out]
      n175 = call-poly "IMAQ Write File 2"("error in (no error)"=w515, "Image Quality"=u32 1000, "File Path"=w517, "Image"=w516) -> ("error out"=w514:errorcluster)  [unwired: 6 in, 1 out]
    }
  }
  "error out" <- w53
